vi "buildTerminalName.vi"(8 "error in (no error)":errorcluster, 9 "Local Terminal Name":string, 10 "Channel Name":string, 11 "session handle":refnum<k15>) -> (0 "error IO":errorcluster, 2 "Fully Qualified Terminal Name":string, 3 "session handle 2":refnum<k15>)   [LabVIEW 2024, in "devicePowerSequencerCoreLogic.lvlib"]
doc: "This SubVI builds a fully qualified terminal name (such as \"/dev1/Engine0/StartTrigger\") based off of the device name, desired channel and desired local terminal name."
uses:
  devicePowerSequencerCoreLogic.lvlib
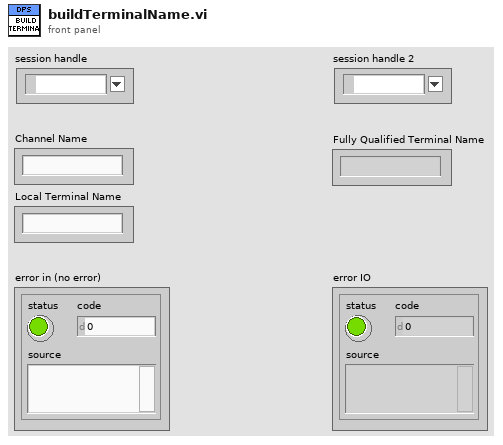
[diagram p1: front panel]
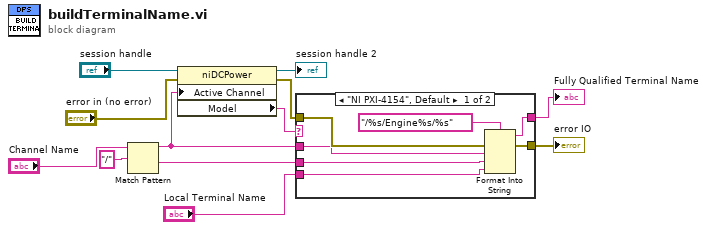
[diagram p0: block diagram]
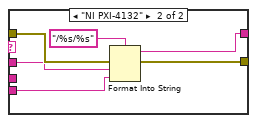
[diagram p2: hidden frame]
diagram:
  n1 = Match Pattern(string="Channel Name", regular expression="/") -> (before substring=w1:string, after substring=w5:string)  [unwired: 1 in, 2 out]
  n2 = property class="niDCPower"(reference="session handle", error in="error in (no error)", "Active Channel"=w1) -> (reference out=→"session handle 2":refnum<k15>, error out=w2:errorcluster, "Model"=w7:string)
  n3 = case shown="\"NI PXI-4154\", Default" w7 {
    tunnel: w2 -> [w19 w25]
    tunnel: [w18 w24] -> w10
    tunnel: [w17 w23] -> w9
    tunnel: "Local Terminal Name" -> [w15 w21]
    tunnel: w1 -> [w14 w20]
    tunnel: w5 -> [w13 _]
    frame "NI PXI-4154", Default {
      n4 = Format Into String(format string="/%s/Engine%s/%s", error in=w19, w14, w13, w15) -> (resulting string=w17:string, error out=w18:errorcluster)  [unwired: 1 in]
    }
    frame "NI PXI-4132" {
      n5 = Format Into String(format string="/%s/%s", error in=w25, w20, w21) -> (resulting string=w23:string, error out=w24:errorcluster)  [unwired: 1 in]
    }
  }
  "error IO" <- w10
  "Fully Qualified Terminal Name" <- w9
